vi "TranslationStageInitDone.vi"(8 "error in (no error)":errorcluster, 10 "Variant":variant, 11 "TranslationStageUI in":refnum<class "TranslationStageUI.lvclass">) -> (0 "error out":errorcluster, 3 "TranslationStageUI out":refnum<class "TranslationStageUI.lvclass">)   [LabVIEW 2023, in "TranslationStage_UI.lvlib" / "TranslationStageUI.lvclass"]
uses:
  TranslationStageUI.lvclass
  TranslationStageUI.lvclass/TranslationStageUI.ctl
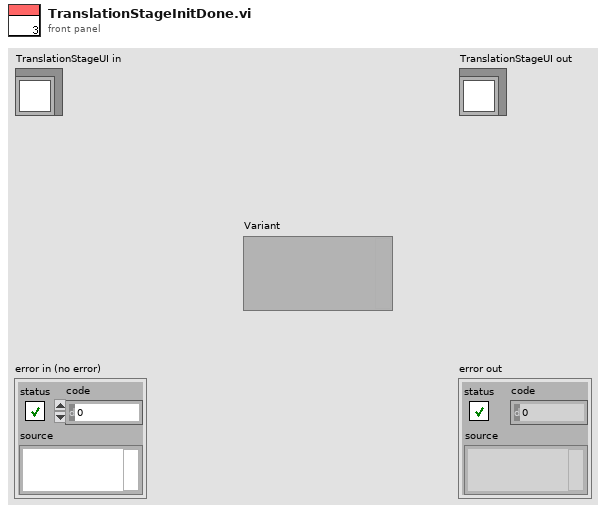
[diagram p1: front panel]
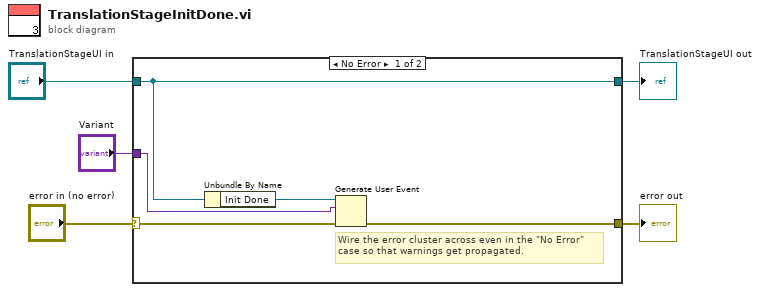
[diagram p0: block diagram]
diagram:
  n1 = case shown="No Error" "error in (no error)" {
    selector: "error in (no error)" -> [w8 w12]
    tunnel: [w7 w12] -> w4
    tunnel: [w9 w11] -> w2
    tunnel: "TranslationStageUI in" -> [w9 w11]
    tunnel: "Variant" -> [w6 _]
    frame No Error {
      # "Wire the error cluster across even in the \"No Error\"\ncase so that warnings get propagated."
      n2 = Unbundle By Name(w9) -> ("Init Done"=w10:refnum<user-event>)
      n3 = Generate User Event(user event=w10, event data cluster=w6, error in=w8) -> (error out=w7:errorcluster)  [unwired: 1 in, 1 out]
    }
    frame Error {
    }
  }
  "error out" <- w4
  "TranslationStageUI out" <- w2
